vi "Trace.vi"(7 "QuWire in":refnum<class "QuWire.lvclass">) -> (8 "Trace":dbl)   [LabVIEW 2020]
uses:
  QuSim/QuWire/QuWire.lvclass
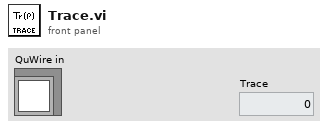
[diagram p1: front panel]
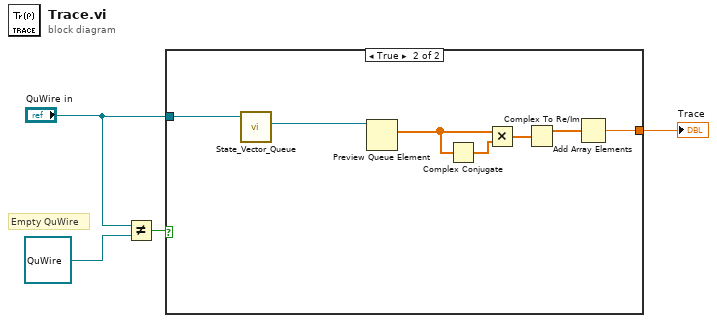
[diagram p0: block diagram]
diagram:
  # "Empty QuWire"
  n1 = Not Equal?(x="QuWire in", y=refnum<class "QuWire.lvclass"> refnum ("QuWire in")) -> (x != y?=w3:bool)
  n2 = case shown="True" w3 {
    tunnel: "QuWire in" -> [_ w7]
    tunnel: [_ w5] -> w1
    frame False {
    }
    frame True {
      n3 = call "State_Vector_Queue.vi"("QuWire in"=w7) -> ("State Vector Queue"=w11:refnum<queue>)  [unwired: 8 in, 2 out]
      n4 = Preview Queue Element(queue=w11) -> (element=w9:cdb[])  [unwired: 2 in, 3 out]
      n5 = Complex Conjugate(1:w9) -> (0:w10:cdb[])
      n6 = Multiply(x=w9, y=w10) -> (x*y=w8:cdb[])
      n7 = Complex To Re/Im(x + iy=w8) -> (x=w6:dbl[])  [unwired: 1 out]
      n8 = Add Array Elements(numeric array=w6) -> (sum=w5:dbl)
    }
  }
  "Trace" <- w1
